vi "GetTestCounter.vi"(7 "Test":T1={"Config"={"Amplification Factor"=2.0, "100% Reflectance Standard"=2.0, "Calculation Method"=enum."Reflectance", "Option to discard new data?"=FALSE, "Mode"=enum."Spectrum", "Number of Averages"=0, "B Test?"=FALSE}, "Indicators"={"DAQ Background Level (V)"=2.0, "A-Test Counter"=2, "B-Test Counter"=2, "Type"=enum."A-Test", "Scope Background Level (Amps)"=2.0, "TAS only?"=FALSE}} {"Config"."Number of Averages" min=0}) -> (3 "Current test counter":i32)   [LabVIEW 2017, in "Scope.lvlib"]
uses:
  Scope.lvlib
  System Control/CTLs/Test params.ctl
  System Control/CTLs/Test Controls.ctl
  System Control/CTLs/Test indicators.ctl
  System Control/CTLs/Test Type.ctl
  System Control/Main controller.lvlib
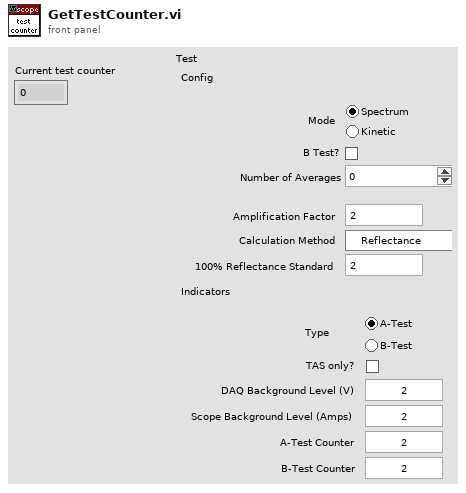
[diagram p1: front panel]
types:
  T1 = typedef "Main controller.lvlib/Test params.ctl" = cluster{"Config":T2, "Indicators":T3}
  T2 = typedef "Main controller.lvlib/Test Controls.ctl" = cluster{"Amplification Factor":dbl, "100% Reflectance Standard":dbl, "Calculation Method":enum16{"Reflectance", "Transmission", "Kubelka-Munk"}, "Option to discard new data?":bool, "Mode":enum32{"Spectrum", "Kinetic"}, "Number of Averages":i32, "B Test?":bool}
  T3 = typedef "Main controller.lvlib/Test indicators.ctl" = cluster{"DAQ Background Level (V)":dbl, "A-Test Counter":i32, "B-Test Counter":i32, "Type":T4, "Scope Background Level (Amps)":dbl, "TAS only?":bool}
  T4 = typedef "Main controller.lvlib/Test Type.ctl" = enum32{"A-Test", "B-Test"}
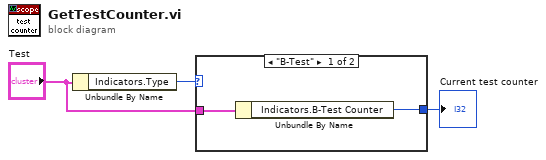
[diagram p0: block diagram]
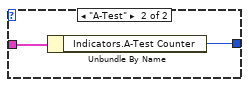
[diagram p2: hidden frame]
diagram:
  n1 = Unbundle By Name("Test") -> ("Indicators.Type"=w2:T4)
  n2 = case shown="\"B-Test\"" w2 {
    tunnel: "Test" -> [w5 w7]
    tunnel: [w4 w6] -> w3
    frame "B-Test" {
      n3 = Unbundle By Name(w5) -> ("Indicators.B-Test Counter"=w4:i32)
    }
    frame "A-Test" {
      n4 = Unbundle By Name(w7) -> ("Indicators.A-Test Counter"=w6:i32)
    }
  }
  "Current test counter" <- w3
